vi "Read Config.vi"(8 "error in (no error)":errorcluster, 9 "Re-Init?":bool, 10 "ICM File In":path, 11 "String Init in":refnum<class "String Init.lvclass">) -> (0 "error out":errorcluster, 3 "String Init out":refnum<class "String Init.lvclass">)   [LabVIEW 2018, in "String Init.lvclass"]
doc: "String Init.lvclass:Read Config.vi\n\nThis VI reads the String Init Class parameters from the ICM configuration file.\n\nInstrument Communication Module Version 1.0\nOctober, 2020 Original Code Consulting Davita Bird\n www.originalcode.com"
uses:
  String Init.lvclass
  String Init.lvclass/String Init.ctl
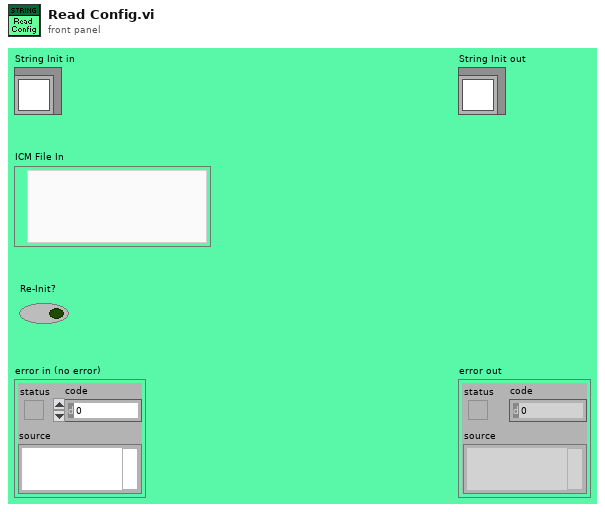
[diagram p1: front panel]
types:
  T1 = typedef "String Init.lvclass/String Init Config.ctl" = cluster{"String":string}
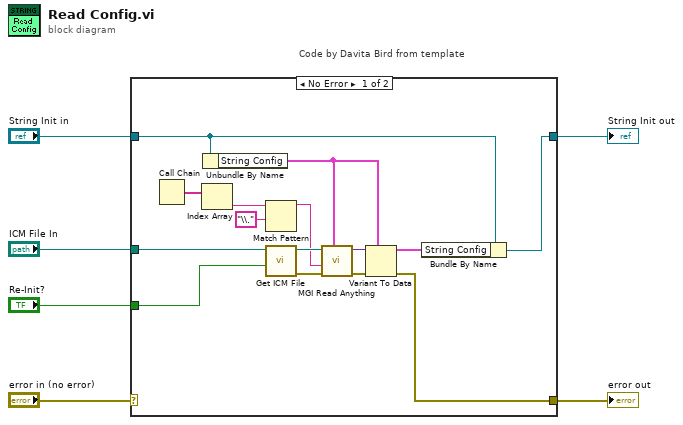
[diagram p0: block diagram]
diagram:
  n1 = case "Code by Davita Bird from template" shown="No Error" "error in (no error)" {
    selector: "error in (no error)" -> [_ w23]
    tunnel: [w13 w23] -> w5
    tunnel: [w10 w22] -> w3
    tunnel: "String Init in" -> [w7 w22]
    tunnel: "ICM File In" -> [w9 _]
    tunnel: "Re-Init?" -> [w8 _]
    frame No Error {
      n2 = Call Chain() -> (call chain=w18:string[])
      n3 = Index Array(array=w18) -> (element=w19:string)  [unwired: 1 in]
      n4 = Unbundle By Name(w7) -> ("String Config"=w11:T1)
      n5 = Match Pattern(string=w19, regular expression="\\.") -> (before substring=w16:string)  [unwired: 1 in, 3 out]
      n6 = call "Get ICM File.vi"("Re-Init?"=w8, "ICM File In"=w9) -> ("error out"=w20:errorcluster, "ICM File"=w21:path)  [unwired: 8 in]
      n7 = call <userlib>:"MGI Read Anything.vi"("Type of Anything"=w11, "Error In"=w20, "Section Name (Name of \"Type of Anything\")"=w16, "Path (dialog)"=w21) -> ("Error Out"=w14:errorcluster, "Anything"=w15:variant)  [unwired: 4 in, 2 out]
      n8 = Variant To Data(error in=w14, type=w11, Variant=w15) -> (data=w12:T1, error out=w13:errorcluster)
      n9 = Bundle By Name(cluster=w7, "String Config"=w12) -> (w10:refnum<class "String Init.lvclass">)
    }
    frame Error {
    }
  }
  "error out" <- w5
  "String Init out" <- w3
